vi "HEX显示.vi"(1 "接收的HEX字符串":string) -> (0 "HEX字符串":string)   [LabVIEW 2020]
panel:
  # "串口接收到HEX数据，通过该vi将HEX数据以字符串正常显示"
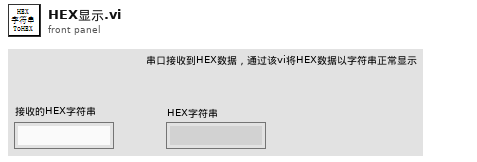
[diagram p1: front panel]
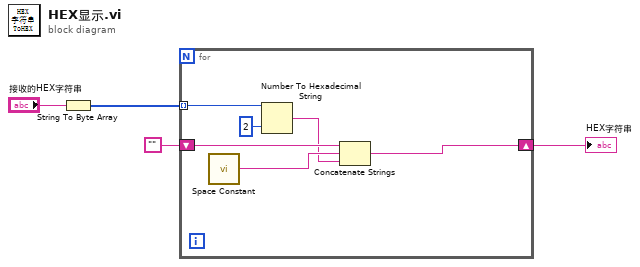
[diagram p0: block diagram]
diagram:
  n1 = String To Byte Array(string="接收的HEX字符串") -> (unsigned byte array=w3:u8[])
  n2 = for {
    tunnel: w3 -> [w10] mode=indexing
    shift-right: [w5] -> w1
    shift-left: "" -> [w8]
    n3 = call <vilib>:"Space Constant.vi"() -> ("String"=w7:string)
    n4 = Number To Hexadecimal String(1:i16 2 ("宽度(-)"), 2:w10) -> (0:w6:string)
    n5 = Concatenate Strings(w8, w7, w6) -> (w5:string)
  }
  "HEX字符串" <- w1
